vi "Element Init.vi"(7 "VolatusAPI":refnum<class "VolatusAPI.lvclass">, 8 "error in (no error)":errorcluster, 10 "JSON":string, 11 "2WayValve in":refnum<class "2WayValveH.lvclass">) -> (0 "error out":errorcluster, 3 "2WayValve out":refnum<class "2WayValveH.lvclass">)   [LabVIEW 2020, in "VolatusGUIElements.lvlib" / "2WayValveH.lvclass"]
uses:
  2WayValveH.lvclass
  C:/dev/lv20CE/relink/lv-volatus/VolatusGUI/GUI Element/GUI Element.lvclass
  Volatus/VolatusAPI/VolatusAPI.lvclass
  JSON.ctl
  Group Channel.ctl
  Unused Element.ctl
  Values.ctl
  Channel State.ctl
  VolatusGUI/GUI Element/GUI Element.lvclass/GUI Element.ctl
  lv-vecto/Vecto/Group DBL/Group DBL.lvclass
  C:/dev/lv20CE/relink/lv-vecto/Vecto/Group/Group.lvclass
  lv-vecto/Vecto/Channel DBL/Channel DBL.lvclass/Channel DBL.ctl
  2WayValveH.lvclass/2WayValveH.ctl
  5ca493e1-1c63-4061-b4b4-46184d61fbe0.vi
  <vilib>/JDP Science/JSONtext/JSON text to Variant.vi
  lv-vecto/Vecto/Group/Channel Info by Index.vi
  <vilib>/JDP Science/JSONtext/LVClass Serializer/JSONtext LVClass Serializer.lvclass
  lv-vecto/Vecto/Channel DBL/Channel DBL.lvclass
  VolatusGUI/Element Inhibit/Element Inhibit.lvclass
  VolatusGUI/GUI Element/GUI Element.lvclass
  VolatusErrorUtilities/MultiErrors/MultiErrors.lvclass
  Volatus/Digital Command/Digital Command.lvclass
  C:/dev/lv20CE/relink/lv-vecto/Vecto/Group DBL/Group DBL.lvclass
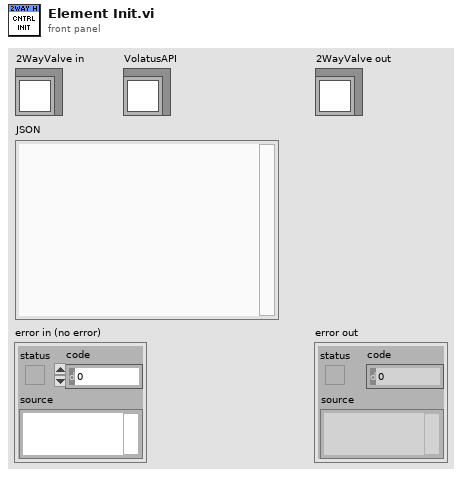
[diagram p1: front panel]
types:
  T1 = typedef "VolatusGUIElements.lvlib/2WayValveH.lvclass/Values.ctl" = cluster{"Command":T2, "CmdFB":T2, "Closed":T2, "Open":T2, "Energized":T2}
  T2 = typedef "VolatusGUIElements.lvlib/2WayValveH.lvclass/Channel State.ctl" = cluster{"Value":bool, "Stale":bool, "Config":bool, "Error":bool, "Prev":bool}
  T3 = typedef "VolatusGUIElements.lvlib/2WayValveH.lvclass/Unused Element.ctl" = cluster{"Command":bool, "Feedback":bool, "Energized":bool}
  T4 = typedef "VolatusGUIElements.lvlib/2WayValveH.lvclass/JSON.ctl" = cluster{"Output":T5, "ClosedFB":T5, "OpenFB":T5, "Energized":cluster{"Channel":string, "Threshold":dbl}, "Staleness":dbl, "Inhibit":string}
  T5 = typedef "VolatusGUIElements.lvlib/2WayValveH.lvclass/Group Channel.ctl" = cluster{"Channel":string}
  T6 = typedef "VectoConfig.lvlib/Channel Info.ctl" = cluster{"Name":string, "Group":string, "Owning Node":string, "Owning Task":string, "Resource":string}
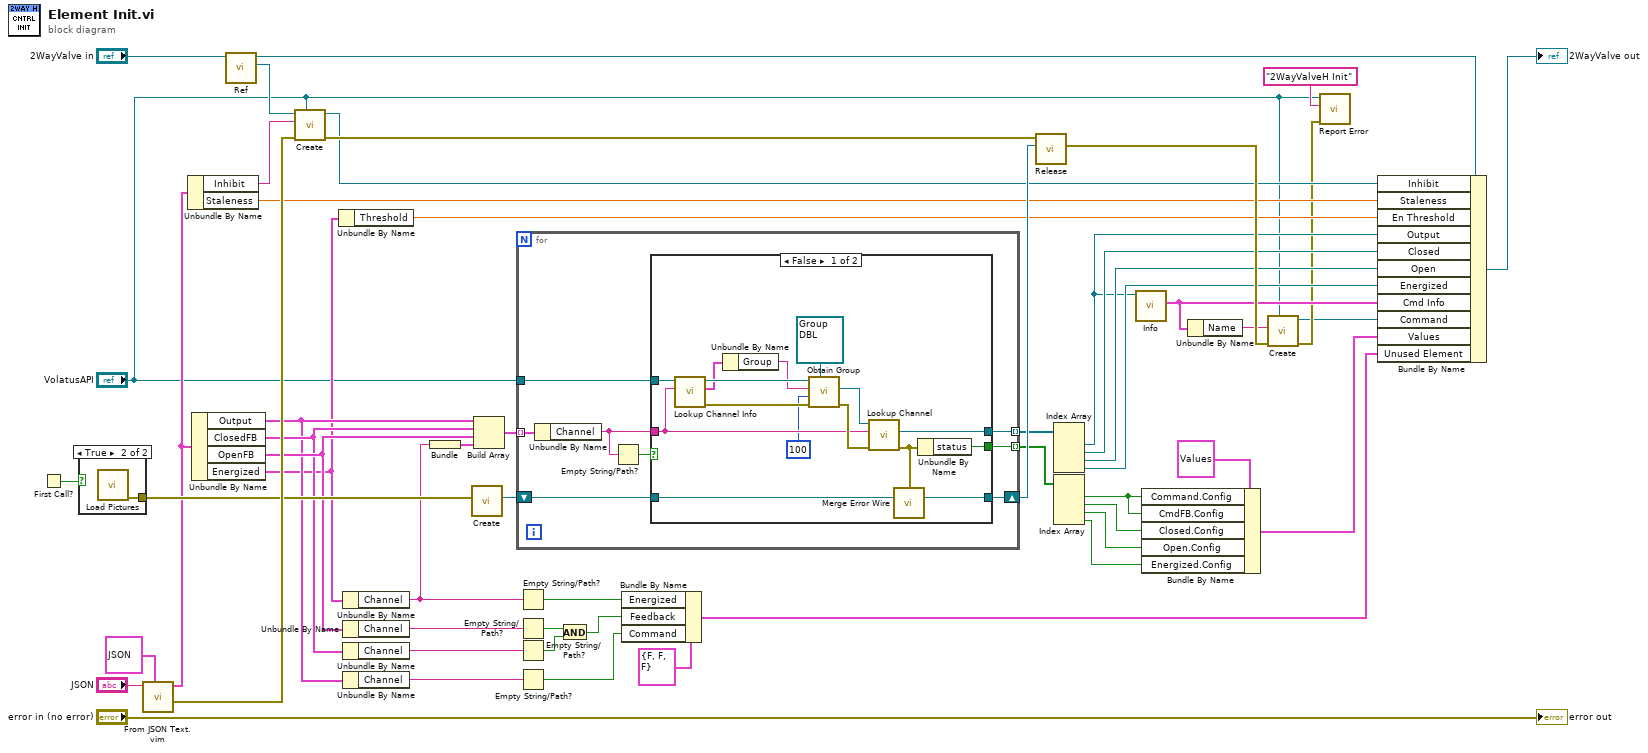
[diagram p0: block diagram]
diagram:
  n1 = First Call?() -> (First Call?: T/F=w22:bool)
  n2 = case shown="True" w22 {
    tunnel: [_ w55] -> w51
    frame False {
    }
    frame True {
      n3 = call "Load Pictures.vi"() -> ("error out"=w55:errorcluster)  [unwired: 11 in]
    }
  }
  n4 = call "From JSON Text.vim"("Data Type and Default Value"=T4 {"Output"={"Channel"=""}, "ClosedFB"={"Channel"=""}, "OpenFB"={"Channel"=""}, "Energized"={"Channel"="", "Threshold"=0.0}, "Staleness"=0.0, "Inhibit"=""} ("JSON"), "JSON"="JSON") -> ("error out"=w53:errorcluster, "Data out"=w15:T4)  [unwired: 8 in]
  n5 = Unbundle By Name(w15) -> ("Inhibit"=w14:string, "Staleness"=w13:dbl)
  n6 = Unbundle By Name(w15) -> ("Output"=w21:T5, "ClosedFB"=w47:T5, "OpenFB"=w48:T5, "Energized"=w17:cluster{"Channel":string, "Threshold":dbl})
  n7 = call "Ref.vi"("GUI Element in"="2WayValve in") -> ("Ref"=w11:refnum<vi>, "GUI Element out"=w12:refnum<class "2WayValveH.lvclass">)  [unwired: 9 in]
  n8 = call "Create.vi"("VolatusAPI"="VolatusAPI", "error in (no error)"=w53, "Inhibit Channel"=w14, "Control Ref"=w11) -> ("error out"=w9:errorcluster, "Element Inhibit out"=w6:refnum<class "Element Inhibit.lvclass">)  [unwired: 6 in]
  n9 = Unbundle By Name(w17) -> ("Threshold"=w16:dbl)
  n10 = Unbundle By Name(w17) -> ("Channel"=w19:string)
  n11 = Unbundle By Name(w48) -> ("Channel"=w46:string)
  n12 = Unbundle By Name(w47) -> ("Channel"=w45:string)
  n13 = Unbundle By Name(w21) -> ("Channel"=w44:string)
  n14 = Bundle("Channel"=w19) -> (w18:cluster{"Channel":string})  [unwired: 1 in]
  n15 = call "Create.vi"("error in (no error)"=w51) -> ("MultiErrors out"=w10:refnum<class "MultiErrors.lvclass">)  [unwired: 10 in]
  n16 = Build Array(w21, w47, w48, w18) -> (w37:T5[])
  n17 = for {
    tunnel: w37 -> [w62] mode=indexing
    tunnel: [w61] -> w36 mode=indexing
    tunnel: [w60] -> w35 mode=indexing
    tunnel: "VolatusAPI" -> [w63]
    shift-right: [w56] -> w52
    shift-left: w10 -> [w57]
    n18 = Unbundle By Name(w62) -> ("Channel"=w59:string)
    n19 = Empty String/Path?(string/path=w59) -> (empty?=w58:bool)
    n20 = case shown="False" w58 {
      tunnel: w63 -> [w77 _]
      tunnel: [w76 _] -> w61
      tunnel: [w75 _] -> w60
      tunnel: w59 -> [w71 _]
      tunnel: w57 -> [w70 w79]
      tunnel: [w65 w79] -> w56
      frame False {
        n21 = call "Lookup Channel Info.vi"("Channel Name"=w71, "VolatusAPI in"=w77) -> ("error out"=w66:errorcluster, "Channel Info"=w73:T6, "VolatusAPI out"=w74:refnum<class "VolatusAPI.lvclass">)  [unwired: 6 in, 1 out]
        n22 = Unbundle By Name(w73) -> ("Group"=w72:string)
        n23 = call "Obtain Group.vi"("Group Type (Abstract)"=refnum<class "Group DBL.lvclass"> refnum ("Vecto.lvlib:Group.lvclass"), "error in (no error)"=w66, "Timeout ms (5000)"=u32 100, "Group Name"=w72, "VolatusAPI in"=w74) -> ("error out"=w78:errorcluster, "Group"=w67:refnum<class "Group DBL.lvclass">)  [unwired: 4 in, 1 out]
        n24 = call "Lookup Channel.vi"("error in (no error)"=w78, "Channel Name"=w71, "Group in"=w67) -> ("error out"=w69:errorcluster, "Channel"=w76:refnum<class "Channel DBL.lvclass">)  [unwired: 6 in, 1 out]
        n25 = call "Merge Error Wire.vi"("error in (no error)"=w69, "MultiErrors in"=w70) -> ("MultiErrors out"=w65:refnum<class "MultiErrors.lvclass">)  [unwired: 13 in]
        n26 = Unbundle By Name(w69) -> ("status"=w75:bool)
      }
      frame True {
      }
    }
  }
  n27 = Empty String/Path?(string/path=w19) -> (empty?=w42:bool)
  n28 = Empty String/Path?(string/path=w46) -> (empty?=w41:bool)
  n29 = Empty String/Path?(string/path=w45) -> (empty?=w40:bool)
  n30 = Empty String/Path?(string/path=w44) -> (empty?=w38:bool)
  n31 = And(x=w41, y=w40) -> (x .and. y?=w39:bool)
  n32 = Bundle By Name(cluster=T3 {"Command"=FALSE, "Feedback"=FALSE, "Energized"=FALSE} ("Unused Element"), "Energized"=w42, "Feedback"=w39, "Command"=w38) -> (w25:T3)
  n33 = call "Release.vi"("MultiErrors in"=w52, "Upstream Error (None)"=w9) -> ("error out"=w54:errorcluster)  [unwired: 9 in]
  n34 = Index Array(array=w36) -> (element #1=w20:refnum<class "Channel DBL.lvclass">, element #2=w29:refnum<class "Channel DBL.lvclass">, element #3=w28:refnum<class "Channel DBL.lvclass">, element #4=w27:refnum<class "Channel DBL.lvclass">)  [unwired: 4 in]
  n35 = Index Array(array=w35) -> (element #1=w33:bool, element #2=w32:bool, element #3=w31:bool, element #4=w30:bool)  [unwired: 4 in]
  n36 = call "Info.vi"("Channel in"=w20) -> ("Info"=w5:T6)  [unwired: 8 in, 2 out]
  n37 = Bundle By Name(cluster=T1 {"Command"={"Value"=FALSE, "Stale"=FALSE, "Config"=FALSE, "Error"=FALSE, "Prev"=FALSE}, "CmdFB"={"Value"=FALSE, "Stale"=FALSE, "Config"=FALSE, "Error"=FALSE, "Prev"=FALSE}, "Closed"={"Value"=FALSE, "Stale"=FALSE, "Config"=FALSE, "Error"=FALSE, "Prev"=FALSE}, "Open"={"Value"=FALSE, "Stale"=FALSE, "Config"=FALSE, "Error"=FALSE, "Prev"=FALSE}, "Energized"={"Value"=FALSE, "Stale"=FALSE, "Config"=FALSE, "Error"=FALSE, "Prev"=FALSE}} ("Values"), "Command.Config"=w33, "CmdFB.Config"=w33, "Closed.Config"=w32, "Open.Config"=w31, "Energized.Config"=w30) -> (w26:T1)
  n38 = Unbundle By Name(w5) -> ("Name"=w4:string)
  n39 = call "Create.vi"("VolatusAPI"="VolatusAPI", "error in (no error)"=w54, "Channel"=w4) -> ("error out"=w2:errorcluster, "Digital Command out"=w1:refnum<class "Digital Command.lvclass">)  [unwired: 7 in]
  n40 = call "Report Error.vi"("error in (no error)"=w2, "Context"="2WayValveH Init", "VolatusAPI in"="VolatusAPI") -> ()  [unwired: 7 in, 2 out]
  n41 = Bundle By Name(cluster=w12, "Inhibit"=w6, "Staleness"=w13, "En Threshold"=w16, "Output"=w20, "Closed"=w29, "Open"=w28, "Energized"=w27, "Cmd Info"=w5, "Command"=w1, "Values"=w26, "Unused Element"=w25) -> (→"2WayValve out":refnum<class "2WayValveH.lvclass">)
  "error out" <- "error in (no error)"
